vi "Horizontal Bar Pictures.vi"() -> (3 "Horizontal bar map":T1)   [LabVIEW 2020, in "BetterDragAndDrop.lvlib" / "BetterHorizontalBar.lvclass"]
uses:
  BetterHorizontalBar.lvclass
  Horizontal Bar Map.ctl
  Horizontal Bar Enumeration.ctl
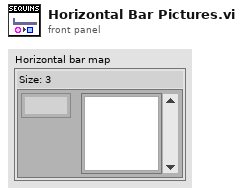
[diagram p1: front panel]
types:
  T1 = typedef "BetterDragAndDrop.lvlib/BetterHorizontalBar.lvclass/Horizontal Bar Map.ctl" = map{T2, picture}
  T2 = typedef "BetterDragAndDrop.lvlib/BetterHorizontalBar.lvclass/Horizontal Bar Enumeration.ctl" = enum16{"None", "only bar", "tilda up"}
  T3 = cluster{"Width":i16, "Style":enum32{"Solid", "Dash", "Dot", "DashDot", "DashDotDot"}}
  T4 = cluster{"left":i16, "top":i16, "right":i16, "bottom":i16}
  T5 = enum32{"Solid", "Dash", "Dot", "DashDot", "DashDotDot"}
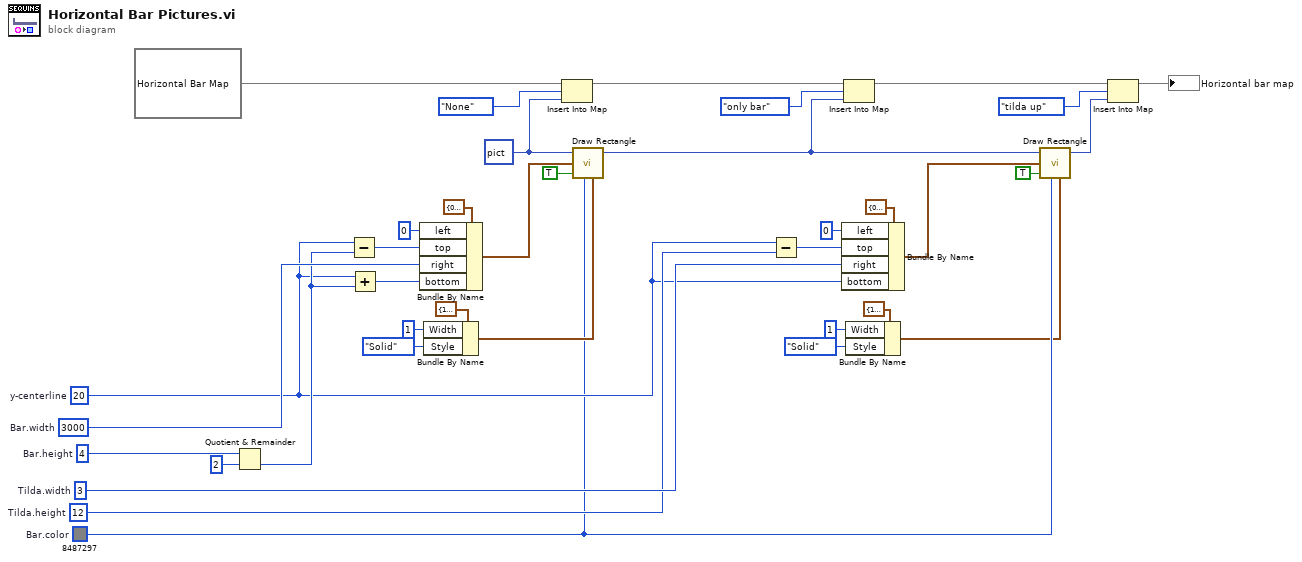
[diagram p0: block diagram]
diagram:
  w31 = i16 3000  # Bar.width
  w20 = i16 12  # Tilda.height
  w21 = i16 3  # Tilda.width
  w30 = i16 4  # Bar.height
  w19 = i16 20  # y-centerline
  w9 = picture data[5B] ("picture")
  w16 = u32 8487297  # Bar.color
  n1 = Quotient & Remainder(x=w30, y=i16 2) -> (floor(x/y)=w28:i16)  [unwired: 1 out]
  n2 = Subtract(x=w19, y=w28) -> (x-y=w26:i16)
  n3 = Add(x=w19, y=w28) -> (x+y=w27:i16)
  n4 = Bundle By Name(cluster=T4 {"left"=0, "top"=0, "right"=0, "bottom"=0} ("rect"), "left"=i16 0, "top"=w26, "right"=w31, "bottom"=w27) -> (w34:T4)
  n5 = Bundle By Name(cluster=T3 {"Width"=1, "Style"=enum."Solid"} ("pen"), "Width"=i16 1, "Style"=T5."Solid") -> (w36:T3)
  n6 = Insert Into Map(map in=T1 {}, key=Horizontal_Bar_Enumeration."None" ("Enum"), value=w9) -> (map out=w7:T1)  [unwired: 2 out]
  n7 = call <vilib>:"Draw Rectangle.vi"("picture"=w9, "rect"=w34, "fill?(F)"=TRUE, "color(black)"=w16, "pen"=w36) -> ("new picture"=w6:picture)  [unwired: 4 in]
  n8 = Subtract(x=w19, y=w20) -> (x-y=w25:i16)
  n9 = Bundle By Name(cluster=T4 {"left"=0, "top"=0, "right"=0, "bottom"=0} ("rect"), "left"=i16 0, "top"=w25, "right"=w21, "bottom"=w19) -> (w18:T4)
  n10 = Insert Into Map(map in=w7, key=Horizontal_Bar_Enumeration."only bar" ("Enum"), value=w6) -> (map out=w4:T1)  [unwired: 2 out]
  n11 = Bundle By Name(cluster=T3 {"Width"=1, "Style"=enum."Solid"} ("pen"), "Width"=i16 1, "Style"=T5."Solid") -> (w11:T3)
  n12 = call <vilib>:"Draw Rectangle.vi"("picture"=w6, "rect"=w18, "fill?(F)"=TRUE, "color(black)"=w16, "pen"=w11) -> ("new picture"=w3:picture)  [unwired: 4 in]
  n13 = Insert Into Map(map in=w4, key=Horizontal_Bar_Enumeration."tilda up" ("Enum"), value=w3) -> (map out=→"Horizontal bar map":T1)  [unwired: 2 out]
